vi "test_TrajectoryAN1106117SinglePoint.vi"   [LabVIEW 2010, in "TrajectoryAN1106117SinglePoint.lvclass"]
uses:
  TrajectoryAN1106117SinglePoint.lvclass
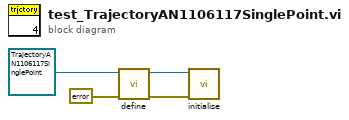
[diagram p0: block diagram]
diagram:
  n1 = call-dynamic "define.vi"("error in (no error)"=errorcluster {"status"=FALSE, "code"=0, "source"=""}, "TrajectoryAN1106117SinglePoint in"=refnum<class "TrajectoryAN1106117SinglePoint.lvclass"> refnum ("TrajectoryAN1106117SinglePoint.lvclass")) -> ("error out"=w2:errorcluster, "TrajectoryAN1106117SinglePoint out"=w1:refnum<class "TrajectoryAN1106117SinglePoint.lvclass">)  [unwired: 8 in]
  n2 = call-dynamic "initialise.vi"("error in (no error)"=w2, "TrajectoryAN1106117SinglePoint in"=w1) -> ()  [unwired: 8 in, 2 out]
